vi "Read Device Information.vi"(8 "error in (no error)":errorcluster, 11 "HFP Gen in":refnum<class "PL HFP Generator.lvclass">) -> (0 "error out":errorcluster, 2 "information":T1, 3 "HFP Gen out":refnum<class "PL HFP Generator.lvclass">)   [LabVIEW 2015, in "PL HFP Generator.lvclass"]
doc: "Reads device information."
uses:
  PL HFP Generator.lvclass
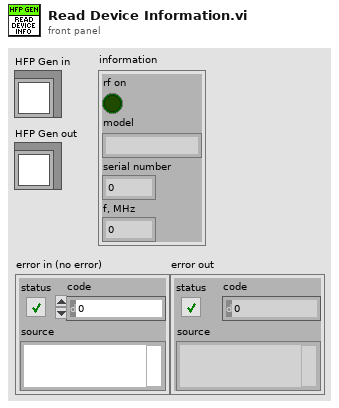
[diagram p1: front panel]
types:
  T1 = cluster{"rf on":bool, "model":string, "serial number":u16, "f, MHz":dbl}
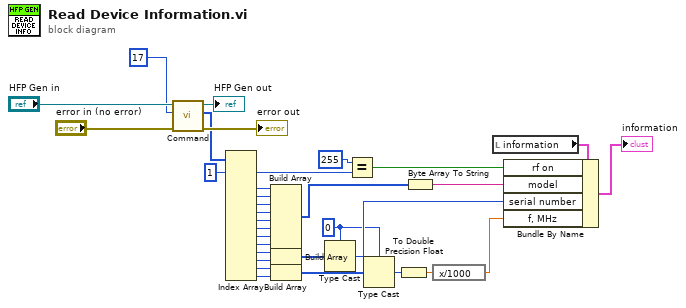
[diagram p0: block diagram]
diagram:
  w8 = u16 0 ("y")
  n1 = call-dynamic "Command.vi"("error in (no error)"="error in (no error)", "function code"=u8 17 ("address"), "MODBUS in"="HFP Gen in") -> ("error out"=→"error out":errorcluster, "data out"=w28:u8[], "MODBUS out"=→"HFP Gen out":refnum<class "PL HFP Generator.lvclass">)  [unwired: 6 in]
  n2 = Index Array(array=w28, index #1=1 ("index")) -> (element #1=w4:u8, element #3=w23:u8, element #4=w22:u8, element #5=w21:u8, element #6=w20:u8, element #7=w19:u8, element #8=w18:u8, element #9=w17:u8, element #10=w16:u8, element #11=w15:u8, element #12=w14:u8, element #13=w11:u8, element #14=w10:u8)  [unwired: 13 in, 1 out]
  n3 = Build Array(w23, w22, w21, w20, w19, w18, w17, w16) -> (w2:u8[])
  n4 = Build Array(w15, w14) -> (w13:u8[])
  n5 = Build Array(w11, w10) -> (w9:u8[])
  n6 = Type Cast(type=w8, x=w13) -> (*(type *) &x=w12:u16)
  n7 = Equal?(x=u8 255 ("y"), y=w4) -> (x = y?=w24:bool)
  n8 = Type Cast(type=w8, x=w9) -> (*(type *) &x=w7:u16)
  n9 = To Double Precision Float(number=w7) -> (double precision float=w6:dbl)
  n10 = Byte Array To String(unsigned byte array=w2) -> (string=w1:string)
  n11 = expression code="x/1000"(w6) -> (w5:dbl)
  n12 = local read "information"() -> (w26:T1)
  n13 = Bundle By Name(cluster=w26, "rf on"=w24, "model"=w1, "serial number"=w12, "f, MHz"=w5) -> (→"information":T1)
